vi "Dresser DXD Get Mode Example.vi"(0 "VISA session":refnum<visa-resource-name>, 5 "DXD Address (1)":T3=1 min=1 max=99 step=1, 11 "Error In (no error)":errorcluster) -> (1 "Mode Byte":u8 format="%.0b", 2 "Bit 0 - Calibration Bit":enum16{"Normal", "Self Cal Mode"}(ring), 3 "Bit 1 - Error Status Character":enum16{"ACK/NAK", "A/N"}(ring), 4 "dup VISA session":refnum<visa-resource-name>, 6 "Bit 2 - End of Line Terminator":enum16{"<cr><lf>", "<cr>"}(ring), 8 "Bit 3 - Echo Bit":enum16{"Command not echoed", "Command returned"}(ring), 10 "Bit 4 - Command Set Bit":enum16{"DXD command set", "ATS command set"}(ring), 12 "Bit 7 - Ad Noise Test Bit":T1(ring), 13 "Bit 6 - Free":enum16{"Free"}(ring), 14 "Bit 5 - Error Status Character":T2(ring)=enum."No error status character (legacy mode)", 15 "Error Out":errorcluster)   [LabVIEW 2015]
doc: "This application example VI demonstrates how to get the Mode of the Dresser DXD Series pressure transducer at the specified address. The initialize and close VI's need to be added to make this VI usable - See Dresser DXD Get and Set Mode.vi\n\nBIT MODE BYTE\n0 Calibration Bit 0=normal 1=self cal mode\n1 Error Status Character 0=ACK/NAK 1=A/N\n2 End of Line Terminator 0=<cr><lf> 1=<cr> (used in DXD Mode only)\n3 Echo Bit 0=command not echoed 1=command returned \n4 Command Set Bit ATS mode select\n5 Error Status Character 1=no error status character. (legacy mode) this overrides bit 1\n 0=Error status character set in bit 1 is returned.\n6 Free\n7 ad noise test bit 0=noise test not performed 1=noise test performed\n\n(Factory default setting of MODE Byte = \"00000000\")\n\n\nWritten by:\nBLOOMY CONTROLS, INC\nWINDSOR, CT 06095, USA\n860-298-9925\nwww.bloomy.com\nV2.0.0\nMay, 2002"
uses:
  Type Defs/DXD Address.ctl
panel:
  # "For instructions on the use of this VI, press Ctrl+H to display the help window and move the mouse over the icon, controls, and indicators"
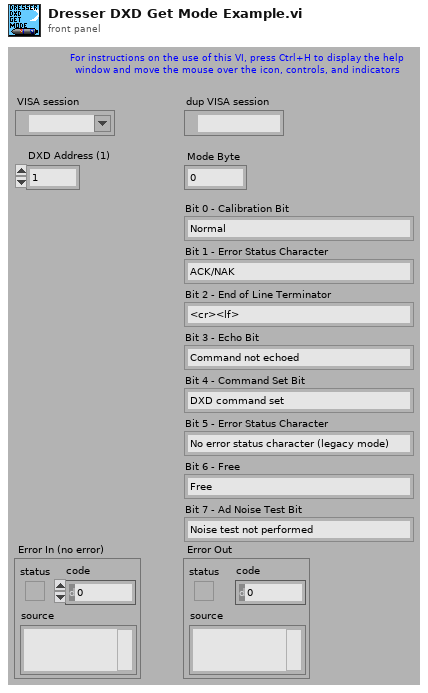
[diagram p1: front panel]
types:
  T1 = enum16{"Noise test not performed", "Noise test performed"}
  T2 = enum16{"Error status character set in bit 1 is returned", "No error status character (legacy mode)"}
  T3 = typedef "DXD Address.ctl" = i32
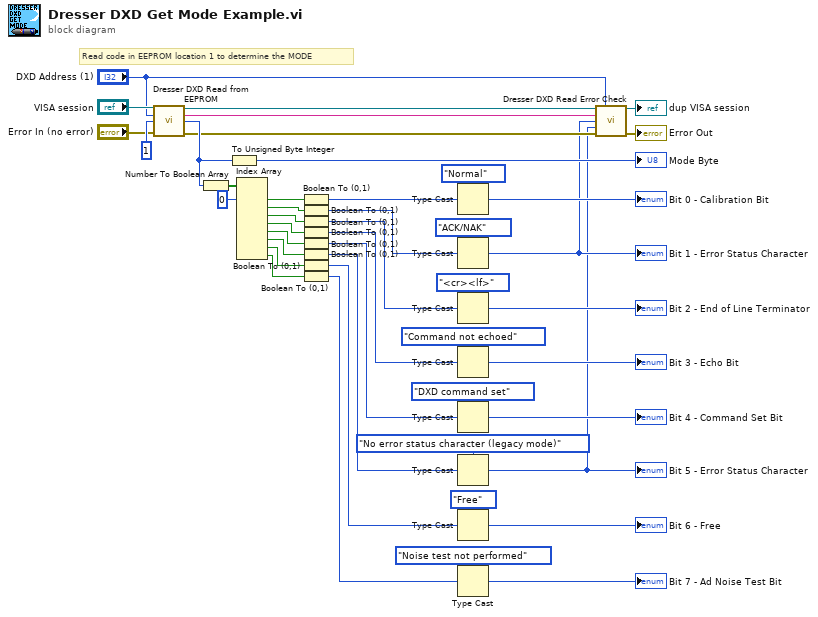
[diagram p0: block diagram]
diagram:
  # "Read code in EEPROM location 1 to determine the MODE"
  n1 = call "Dresser DXD Read from EEPROM.vi"("VISA session"="VISA session", "DXD Address (1)"="DXD Address (1)", "EEPROM Read Address (0)"=1 ("EEPROM Read Address"), "Error In (no error)"="Error In (no error)") -> ("dup VISA session"=w8:refnum<visa-resource-name>, "Returned String"=w6:string, "EEPROM Value"=w9:i32, "Error Out"=w7:errorcluster)  [unwired: 8 in]
  n2 = Number To Boolean Array(number=w9) -> (Boolean array=w29:bool[])
  n3 = To Unsigned Byte Integer(number=w9) -> (unsigned 8bit integer=→"Mode Byte":u8)
  n4 = Index Array(array=w29, index #1=0 ("Index")) -> (element #1=w25:bool, element #2=w26:bool, element #3=w24:bool, element #4=w20:bool, element #5=w21:bool, element #6=w22:bool, element #7=w23:bool, element #8=w19:bool)  [unwired: 7 in]
  n5 = Boolean To (0,1)(Boolean=w25) -> (0, 1=w18:i16)
  n6 = Boolean To (0,1)(Boolean=w26) -> (0, 1=w16:i16)
  n7 = Boolean To (0,1)(Boolean=w24) -> (0, 1=w15:i16)
  n8 = Boolean To (0,1)(Boolean=w20) -> (0, 1=w14:i16)
  n9 = Boolean To (0,1)(Boolean=w21) -> (0, 1=w13:i16)
  n10 = Boolean To (0,1)(Boolean=w22) -> (0, 1=w12:i16)
  n11 = Boolean To (0,1)(Boolean=w23) -> (0, 1=w11:i16)
  n12 = Boolean To (0,1)(Boolean=w19) -> (0, 1=w10:i16)
  n13 = Type Cast(type=enum16{"Normal", "Self Cal Mode"}."Normal" ("Bit 0 - Calibration Bit"), x=w18) -> (*(type *) &x=→"Bit 0 - Calibration Bit":enum16{"Normal", "Self Cal Mode"})
  n14 = Type Cast(type=enum16{"ACK/NAK", "A/N"}."ACK/NAK" ("Bit 1 - Error Status Character"), x=w16) -> (*(type *) &x=w2:enum16{"ACK/NAK", "A/N"})
  "Bit 1 - Error Status Character" <- w2
  n15 = Type Cast(type=enum16{"<cr><lf>", "<cr>"}."<cr><lf>" ("Bit 2 - End of Line Terminator"), x=w15) -> (*(type *) &x=→"Bit 2 - End of Line Terminator":enum16{"<cr><lf>", "<cr>"})
  n16 = Type Cast(type=enum16{"Command not echoed", "Command returned"}."Command not echoed" ("Bit 3 - Echo Bit"), x=w14) -> (*(type *) &x=→"Bit 3 - Echo Bit":enum16{"Command not echoed", "Command returned"})
  n17 = Type Cast(type=enum16{"DXD command set", "ATS command set"}."DXD command set" ("Bit 4 - Command Set Bit"), x=w13) -> (*(type *) &x=→"Bit 4 - Command Set Bit":enum16{"DXD command set", "ATS command set"})
  n18 = Type Cast(type=T2."No error status character (legacy mode)" ("Bit 5 - Error Status Character"), x=w12) -> (*(type *) &x=w1:T2)
  "Bit 5 - Error Status Character" <- w1
  n19 = Type Cast(type=enum16{"Free"}."Free" ("Bit 6 - Free"), x=w11) -> (*(type *) &x=→"Bit 6 - Free":enum16{"Free"})
  n20 = Type Cast(type=T1."Noise test not performed" ("Bit 7 - Ad Noise Test Bit"), x=w10) -> (*(type *) &x=→"Bit 7 - Ad Noise Test Bit":T1)
  n21 = call "Dresser DXD Read Error Check.vi"("VISA session"=w8, "DXD Address (1)"="DXD Address (1)", "Returned String (\"\")"=w6, "Mode Bit 1 - Error Status Character"=w2, "Mode Bit 5 - Error Status Character"=w1, "Error In (no error)"=w7) -> ("dup VISA session"=→"dup VISA session":refnum<visa-resource-name>, "Error Out"=→"Error Out":errorcluster)  [unwired: 6 in, 2 out]
